vi "Write Steps.vi"(8 "error in (no error)":errorcluster, 10 "Steps":refnum<class "Step.lvclass">[](array[class]), 11 "Parallel Step in":refnum<class "Parallel Step.lvclass">) -> (0 "error out":errorcluster, 3 "Parallel Step out":refnum<class "Parallel Step.lvclass">)   [LabVIEW 2015, in "Parallel Step.lvclass"]
uses:
  Parallel Step.lvclass
  classes/Step/Execution/Step.lvclass
  Parallel Step.lvclass/Parallel Step.ctl
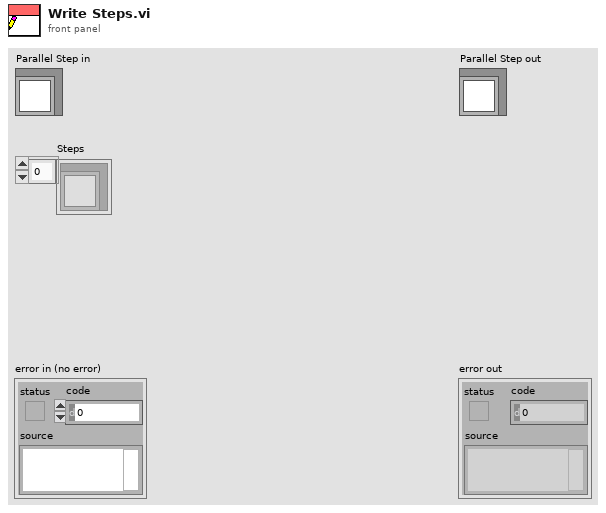
[diagram p1: front panel]
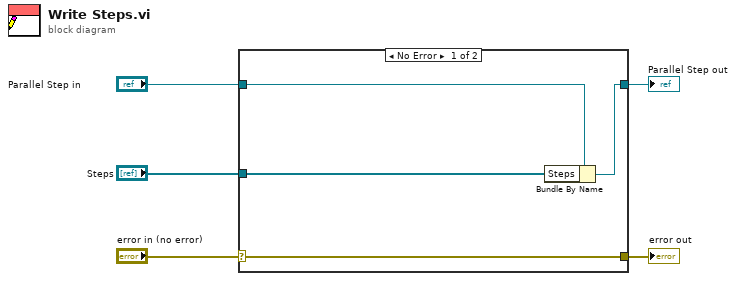
[diagram p0: block diagram]
diagram:
  n1 = case shown="No Error" "error in (no error)" {
    selector: "error in (no error)" -> [w9 w10]
    tunnel: [w9 w10] -> w4
    tunnel: [w7 w11] -> w2
    tunnel: "Parallel Step in" -> [w8 w11]
    tunnel: "Steps" -> [w6 _]
    frame No Error {
      n2 = Bundle By Name(cluster=w8, "Steps"=w6) -> (w7:refnum<class "Parallel Step.lvclass">)
    }
    frame Error {
    }
  }
  "error out" <- w4
  "Parallel Step out" <- w2
